vi "fbg_transform test.vi"() -> ()   [LabVIEW 2013]
uses:
  <vilib>/Analysis/NI_AALBase.lvlib
  <vilib>/Analysis/Matrix/NI_Matrix.lvlib
  <vilib>/Analysis/Matrix/Numeric/Conversions/Array To Matrix - RA2.vi
  <vilib>/Analysis/baseanly.llb/Vector x A.vi
  <vilib>/Analysis/Matrix/Datatypes/RealMatrix.ctl
panel:
  out "FBG Z axis rotation":T1
  in  "Identity":dbl[][](array[numeric])=[[1.0, 0.0, 0.0], [0.0, 1.0, 0.0], [0.0, 0.0, 1.0]]
  in  "Accel Transform":dbl[][](array[numeric])=[[0.7040626542283038, 0.5880062661617681, 0.38499190047152737], [-0.7011382674312465, 0.6254069143025693, 0.32702494518835534], [-0.04873620480650988, -0.5027811258840006, 0.8570355095364262]]
  in  "Output Rotation":dbl[][](array[numeric])
  out "error":dbl[](array[numeric])
  out "FBG Output":dbl[](array[numeric])
  out "FBG tranformed":dbl[](array[numeric])
  in  "FBG Input":dbl[](array[numeric])=[5.0, 2.0, 8.0]
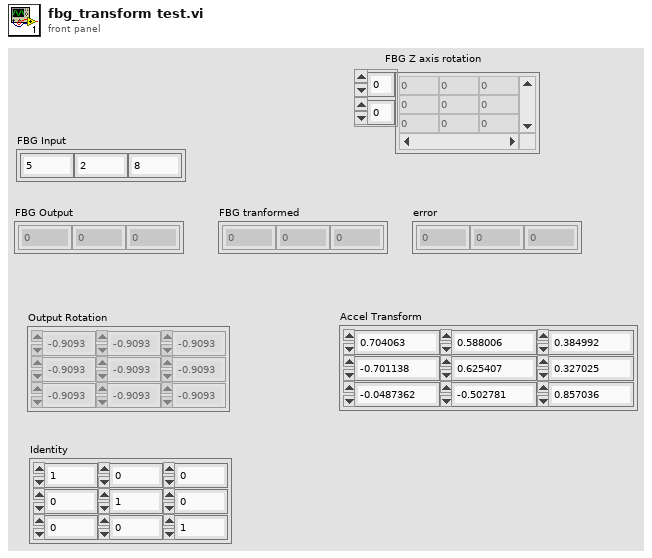
[diagram p1: front panel]
types:
  T1 = typedef "NI_Matrix.lvlib/RealMatrix.ctl" = dbl[][]
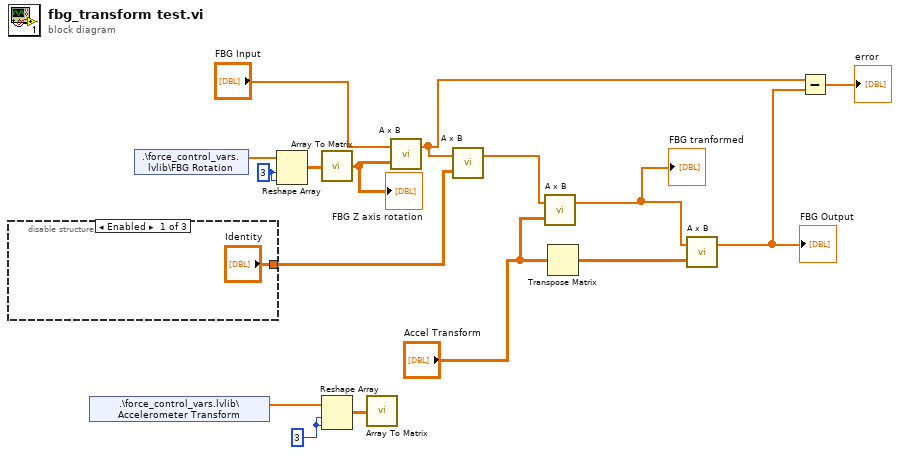
[diagram p0: block diagram]
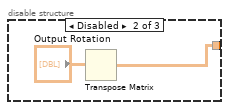
[diagram p2: hidden frame]
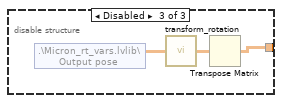
[diagram p3: hidden frame]
diagram:
  w3 = 3 ("dimension size")
  w16 = 3 ("dimension size")
  n1 = disable-structure shown="Enabled" {
    disable-tunnel: ["Identity" w18 w20] -> w13
    frame Enabled {
    }
    frame Disabled {
      n2 = Transpose Matrix(1:"Output Rotation") -> (0:w18:dbl[][])
    }
    frame Disabled {
      n3 = shared-variable ".\\Micron_rt_vars.lvlib\\Output pose"() -> (w22:sgl[][])  [unwired: 1 in, 1 out]
      n4 = call "transform_rotation.vi"("Transform"=w22) -> ("Rotation"=w21:T1)  [unwired: 4 in]
      n5 = Transpose Matrix(1:w21) -> (0:w20:T1)
    }
  }
  n6 = shared-variable ".\\force_control_vars.lvlib\\Accelerometer Transform"() -> (w6:dbl[])  [unwired: 1 in, 1 out]
  n7 = shared-variable ".\\force_control_vars.lvlib\\FBG Rotation"() -> (w2:dbl[])  [unwired: 1 in, 1 out]
  n8 = Reshape Array(w2, w3, w3) -> (w4:dbl[][])
  n9 = call-poly <vilib>:"Array To Matrix.vi"("Real 2D Array"=w4) -> ("Real Matrix"=w1:T1)
  "FBG Z axis rotation" <- w1
  n10 = Reshape Array(w6, w16, w16) -> (w8:dbl[][])
  n11 = call-poly <vilib>:"Array To Matrix.vi"("Real 2D Array"=w8) -> ()  [unwired: 1 out]
  n12 = call-poly <vilib>:"A x B.vi"("Matrix A"=w1, "Vector V'"="FBG Input") -> ("V' x A"=w5:dbl[])  [unwired: 1 out]
  n13 = call-poly <vilib>:"A x B.vi"("Matrix A"=w13, "Vector V'"=w5) -> ("V' x A"=w10:dbl[])  [unwired: 1 out]
  n14 = call-poly <vilib>:"A x B.vi"("Matrix A"="Accel Transform", "Vector V'"=w10) -> ("V' x A"=w12:dbl[])  [unwired: 1 out]
  "FBG tranformed" <- w12
  n15 = Transpose Matrix(1:"Accel Transform") -> (0:w11:dbl[][])
  n16 = call-poly <vilib>:"A x B.vi"("Matrix A"=w11, "Vector V'"=w12) -> ("V' x A"=w15:dbl[])  [unwired: 1 out]
  "FBG Output" <- w15
  n17 = Subtract(x=w5, y=w15) -> (x-y=→"error":dbl[])
